vi "FEA_Model_Sample.vi"(8 "error in (no error)":errorcluster, 9 "include extremes":bool=TRUE, 10 "standard_deviation":dbl, 11 "FEA_Model in":refnum<class "FEA_Model.lvclass">) -> (0 "error out":errorcluster, 3 "FEA_Model out":refnum<class "FEA_Model.lvclass">)   [LabVIEW 2021, in "FEA_Model.lvclass"]
uses:
  FEA_Model.lvclass
  FEA_Model.lvclass/FEA_Model.ctl
  de957b9d-3b39-418b-bf55-63c688e4ea67.vi
  fbdf095a-6d06-4ca0-9642-1e4932d1de12.vi
  <vilib>/gmath/statdist.llb/Normal PDF.vi
  <vilib>/Comparison/Less/Less Functor/Less Functor.lvclass
  <vilib>/gmath/NI_Gmath.lvlib
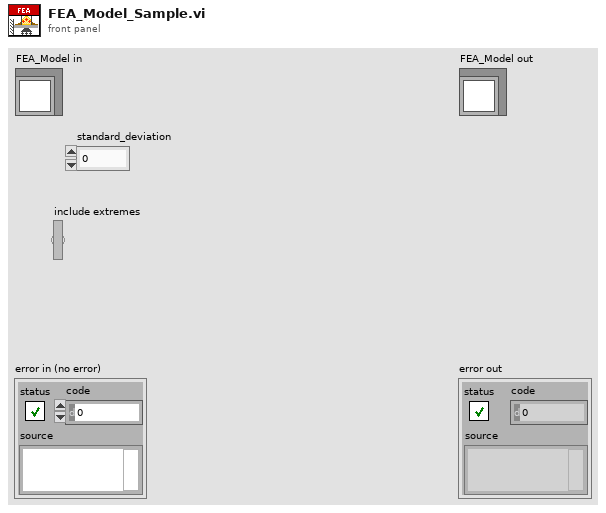
[diagram p1: front panel]
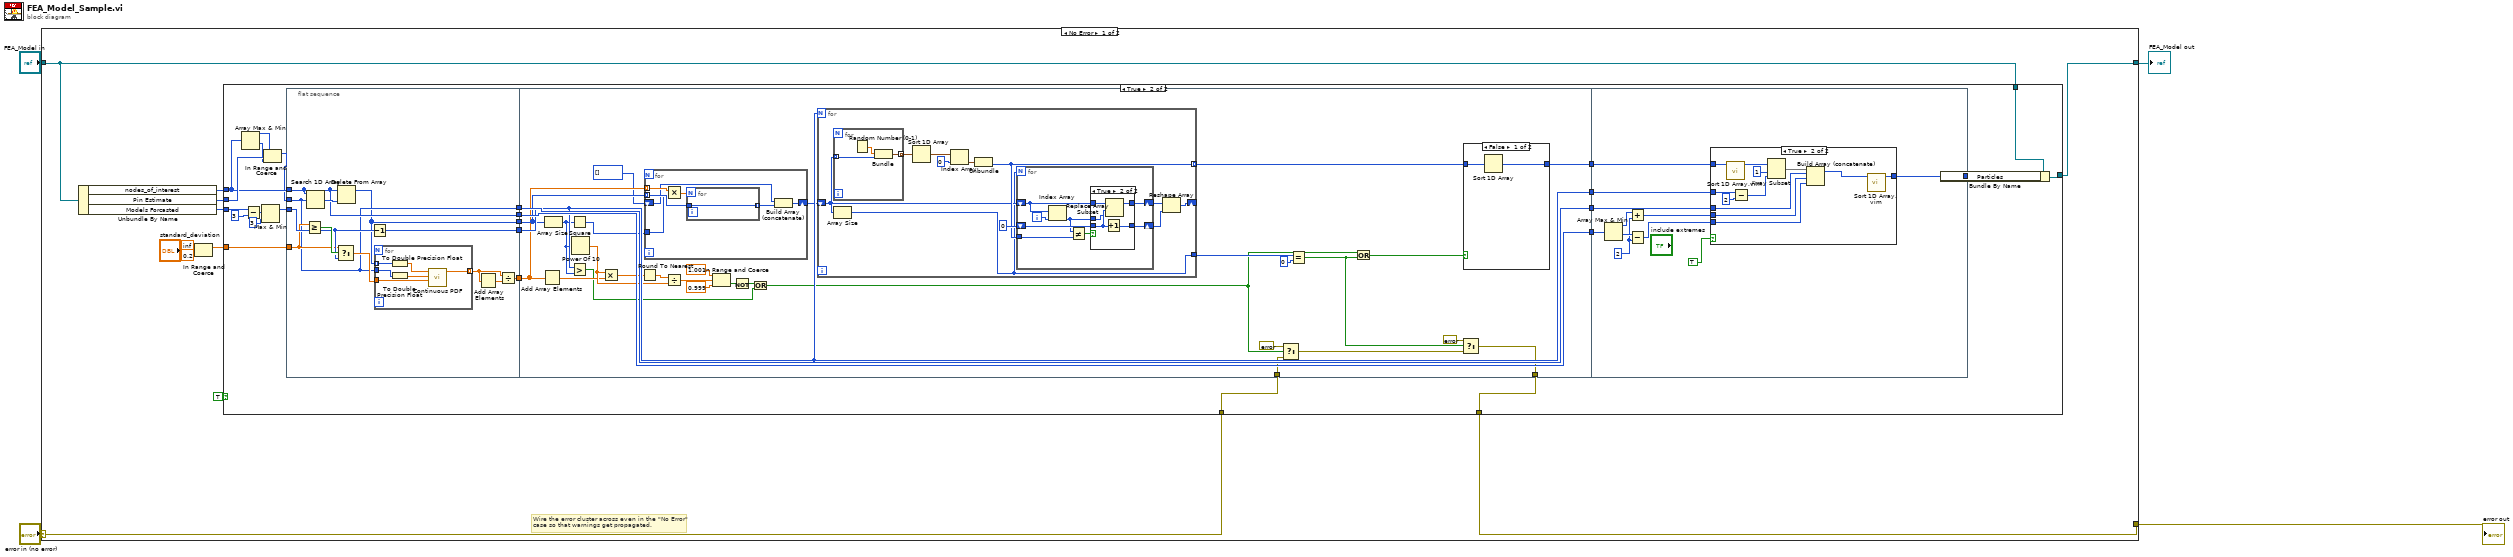
[diagram p0: block diagram]
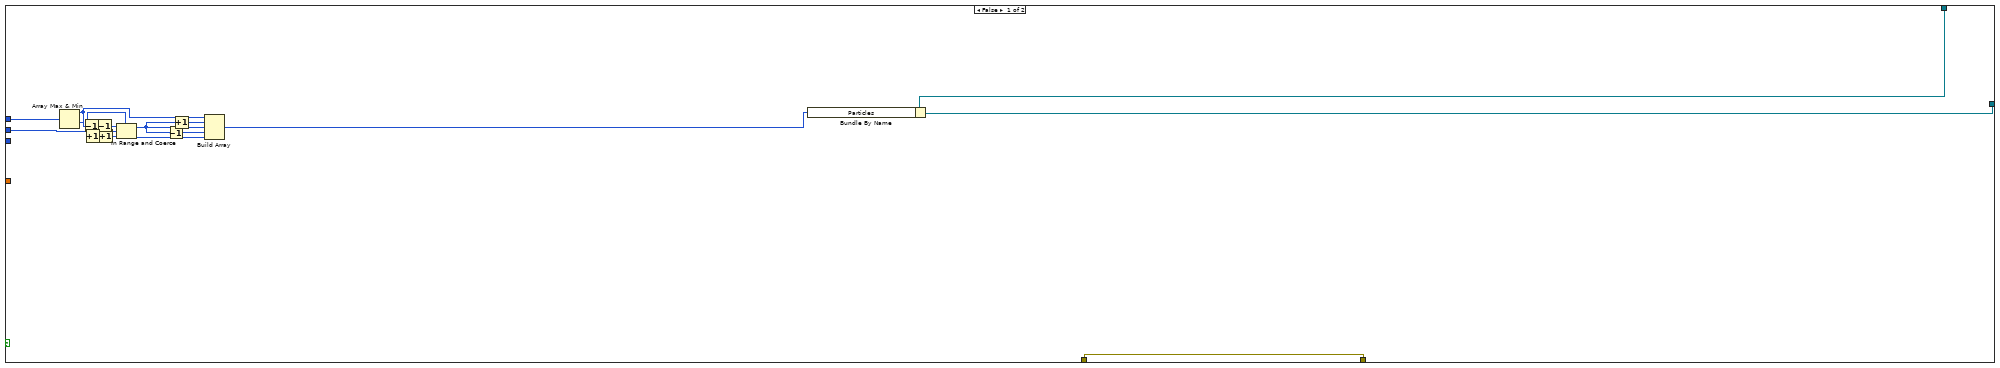
[diagram p2: hidden frame]
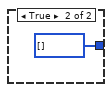
[diagram p3: hidden frame]
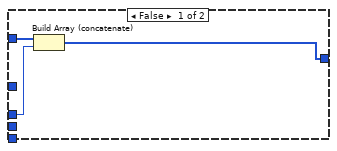
[diagram p5: hidden frame]
diagram:
  n1 = case shown="No Error" "error in (no error)" {
    selector: "error in (no error)" -> [w13 w173]
    tunnel: [w12 w173] -> w3
    tunnel: [w9 w172] -> w1
    tunnel: "FEA_Model in" -> [w10 w172]
    frame No Error {
      # "Wire the error cluster across even in the \"No Error\"\ncase so that warnings get propagated."
      n2 = Unbundle By Name(w10) -> ("nodes_of_interest"=w16:i32[], "Pin Estimate"=w15:i32, "Models Forcasted"=w14:i32)
      n3 = In Range and Coerce(upper limit=inf, x="standard_deviation", lower limit=0.2) -> (coerced(x)=w6:dbl)  [unwired: 1 out]
      n4 = case shown="True" TRUE {
        tunnel: w16 -> [w31 w35]
        tunnel: w15 -> [w27 w36]
        tunnel: w6 -> [_ w47]
        tunnel: [w30 w42] -> w9
        tunnel: w14 -> [_ w41]
        tunnel: w13 -> [w28 w45]
        tunnel: [w28 w44] -> w12
        tunnel: w10 -> [w29 w43]
        frame False {
          n5 = Array Max & Min(array=w31) -> (max value=w25:i32, min value=w24:i32)  [unwired: 2 out]
          n6 = Decrement(x=w25) -> (x-1=w22:i32)
          n7 = Increment(x=w24) -> (x+1=w23:i32)
          n8 = Decrement(x=w22) -> (x-1=w21:i32)
          n9 = Increment(x=w23) -> (x+1=w20:i32)
          n10 = In Range and Coerce(upper limit=w21, x=w27, lower limit=w20) -> (coerced(x)=w19:i32)  [unwired: 1 out]
          n11 = Decrement(x=w19) -> (x-1=w17:i32)
          n12 = Increment(x=w19) -> (x+1=w18:i32)
          n13 = Build Array(w25, w18, w19, w17, w24) -> (w26:i32[])
          n14 = Bundle By Name(cluster=w29, "Particles"=w26) -> (w30:refnum<class "FEA_Model.lvclass">)
        }
        frame True {
          n15 = Array Max & Min(array=w35) -> (max value=w34:i32, min value=w33:i32)  [unwired: 2 out]
          n16 = Subtract(x=w41, y=3) -> (x-y=w40:i32)
          n17 = Max & Min(x=w40, y=3) -> (max(x,y)=w37:i32)  [unwired: 1 out]
          n18 = In Range and Coerce(upper limit=w34, x=w36, lower limit=w33) -> (coerced(x)=w32:i32)  [unwired: 1 out]
          n19 = flat-sequence {
            tunnel: w35 -> [w63]
            tunnel: w32 -> [w60]
            tunnel: [w60] -> w56
            tunnel: [w59] -> w55
            tunnel: [w63] -> w54
            tunnel: [w57] -> w53
            tunnel: [w58] -> w52
            tunnel: w37 -> [w62]
            tunnel: w47 -> [w61]
            tunnel: [w102] -> w51
            tunnel: [w105] -> w50
            tunnel: [w103] -> w49
            tunnel: [w104] -> w48
            tunnel: w56 -> [w105]
            tunnel: w55 -> [w103]
            tunnel: w54 -> [w104]
            tunnel: w53 -> [w101]
            tunnel: w52 -> [w100]
            tunnel: [w76] -> w44
            tunnel: w45 -> [w75]
            tunnel: w51 -> [w156]
            tunnel: w50 -> [w155]
            tunnel: w49 -> [w154]
            tunnel: w48 -> [w153]
            tunnel: [w147] -> w46
            frame #0 {
              n20 = Greater Or Equal?(x=w61, y=w62) -> (x >= y?=w66:bool)
              n21 = Search 1D Array(1D array=w63, element=w60) -> (index of element=w68:i32)  [unwired: 1 in]
              n22 = Select(t=w61, s=w66, f=w62) -> (s? t:f=w67:dbl)
              n23 = Delete From Array(array=w63, index=w68) -> (array with subset deleted=w58:i32[])  [unwired: 1 in, 1 out]
              n24 = Decrement(x=w62) -> (x-1=w59:i32)
              n25 = for {
                tunnel: w58 -> [w71] mode=indexing
                tunnel: [w74] -> w65 mode=indexing
                tunnel: w60 -> [w70]
                tunnel: w67 -> [w73]
                n26 = To Double Precision Float(number=w71) -> (double precision float=w72:dbl)
                n27 = To Double Precision Float(number=w70) -> (double precision float=w69:dbl)
                n28 = call-poly <vilib>:"Continuous PDF.vi"("std"=w73, "mean"=w69, "x"=w72) -> ("pdf(x)"=w74:dbl)  [unwired: 7 in, 1 out]
              }
              n29 = Add Array Elements(numeric array=w65) -> (sum=w64:dbl)
              n30 = Divide(x=w65, y=w64) -> (x/y=w57:dbl[])
            }
            frame #1 {
              n31 = Add Array Elements(numeric array=w101) -> (sum=w90:dbl)
              n32 = Array Size(array=w100) -> (size(s)=w88:i32)
              n33 = Square(x=w88) -> (x^2=w89:i32)
              n34 = Greater?(x=w103, y=w88) -> (0:w87:bool)
              n35 = Power Of 10(x=w88) -> (10^x=w91:dbl)
              n36 = Multiply(x=w91, y=w90) -> (x*y=w93:dbl)
              n37 = Round To Nearest(number=w93) -> (nearest integer value=w92:dbl)
              n38 = for {
                tunnel: w101 -> [w144] mode=indexing
                tunnel: w100 -> [w142] mode=indexing
                shift-right: [w140] -> w85
                shift-left: i32[] [] -> [w139]
                tunnel: w89 -> [w138]
                n39 = Multiply(x=w144, y=w138) -> (x*y=w143:dbl)
                n40 = for {
                  N: w143 -> [_]
                  tunnel: w142 -> [w145]
                  tunnel: [w145] -> w141 mode=indexing
                }
                n41 = Build Array (concatenate)(w139, w141) -> (w140:i32[])
              }
              n42 = Divide(x=w92, y=w91) -> (x/y=w95:dbl)
              n43 = In Range and Coerce(upper limit=1.001, x=w95, lower limit=0.999) -> (In Range?=w98:bool)  [unwired: 1 out]
              n44 = Not(x=w98) -> (.not. x?=w99:bool)
              n45 = Or(x=w99, y=w87) -> (x .or. y?=w77:bool)
              n46 = for {
                N: w103 -> [_]
                tunnel: [w112] -> w80 mode=indexing
                shift-right: [w111] -> _
                shift-left: w85 -> [w110]
                tunnel: [w109] -> w82
                n47 = for {
                  tunnel: [w137] -> w119 mode=indexing
                  tunnel: w110 -> [w135] mode=indexing
                  n48 = Random Number (0-1)() -> (number: 0 to 1=w136:dbl)
                  n49 = Bundle("number: 0 to 1"=w136, w135) -> (w137:cluster{"number: 0 to 1":dbl, i32})  [unwired: 1 out]
                }
                n50 = Array Size(array=w110) -> (size(s)=w109:i32)
                n51 = Sort 1D Array(array=w119) -> (sorted array=w118:cluster{"number: 0 to 1":dbl, i32}[])
                n52 = Index Array(array=w118, index=0) -> (element=w117:cluster{"number: 0 to 1":dbl, i32})
                n53 = Unbundle(w117) -> (w112:i32)  [unwired: 1 out]
                n54 = for {
                  N: w109 -> [_]
                  shift-right: [w127] -> w114
                  shift-left: w110 -> [w125]
                  shift-right: [w123] -> w113
                  shift-left: 0 -> [w124]
                  tunnel: w112 -> [w122]
                  i -> [w126]
                  n55 = Index Array(array=w125, index=w126) -> (element=w120:i32)
                  n56 = Not Equal?(x=w120, y=w122) -> (x != y?=w121:bool)
                  n57 = case shown="True" w121 {
                    tunnel: w125 -> [w129 w134]
                    tunnel: [w129 w133] -> w127
                    tunnel: w124 -> [w128 w132]
                    tunnel: [w128 w131] -> w123
                    tunnel: w120 -> [_ w130]
                    frame False {
                    }
                    frame True {
                      n58 = Increment(x=w132) -> (x+1=w131:i32)
                      n59 = Replace Array Subset(array=w134, new element=w130, index=w132) -> (w133:i32[])
                    }
                  }
                }
                n60 = Reshape Array(w114, w113) -> (w111:i32[])
              }
              n61 = Select(t=errorcluster {"status"=FALSE, "code"=0, "source"="probability not equal to 1"} ("error constant"), s=w77, f=w75) -> (s? t:f=w81:errorcluster)
              n62 = Equal?(x=w82, y=0) -> (x = y?=w79:bool)
              n63 = Or(x=w77, y=w79) -> (x .or. y?=w78:bool)
              n64 = Select(t=errorcluster {"status"=FALSE, "code"=0, "source"="sampled more values than unique numbers"} ("error constant"), s=w79, f=w81) -> (s? t:f=w76:errorcluster)
              n65 = case shown="False" w78 {
                tunnel: [w106 i32[] []] -> w102
                tunnel: w80 -> [w107 _]
                frame False {
                  n66 = Sort 1D Array(array=w107) -> (sorted array=w106:i32[])
                }
                frame True {
                }
              }
            }
            frame #2 {
              w148 = 2 ("y")
              n67 = Array Max & Min(array=w153) -> (max value=w151:i32, min value=w152:i32)  [unwired: 2 out]
              n68 = Add(x=w151, y=w148) -> (x+y=w150:i32)
              n69 = Subtract(x=w152, y=w148) -> (x-y=w149:i32)
              n70 = case shown="True" TRUE ("include extremes") {
                tunnel: w156 -> [w159 w171]
                tunnel: [w157 w163] -> w147
                tunnel: w155 -> [w158 w164]
                tunnel: w150 -> [_ w161]
                tunnel: w149 -> [_ w160]
                tunnel: w154 -> [_ w168]
                frame False {
                  n71 = Build Array (concatenate)(w159, w158) -> (w157:i32[])
                }
                frame True {
                  n72 = call "Sort 1D Array.vim"("unsorted array"=w171) -> ("sorted array"=w170:i32[])  [unwired: 10 in]
                  n73 = Subtract(x=w168, y=2) -> (x-y=w167:i32)
                  n74 = Array Subset(array=w170, index=1, length=w167) -> (w165:i32[])
                  n75 = Build Array (concatenate)(w165, w164, w161, w160) -> (w162:i32[])
                  n76 = call "Sort 1D Array.vim"("unsorted array"=w162) -> ("sorted array"=w163:i32[])  [unwired: 10 in]
                }
              }
            }
          }
          n77 = Bundle By Name(cluster=w43, "Particles"=w46) -> (w42:refnum<class "FEA_Model.lvclass">)
        }
      }
    }
    frame Error {
    }
  }
  "error out" <- w3
  "FEA_Model out" <- w1
